vi "列表.vi"(9 "Bool引用句柄":refnum<vi>, 10 "簇":T4, 11 "事件注册引用句柄 2":refnum<event-registration>) -> ()   [LabVIEW 2020]
uses:
  <vilib>/Utility/miscctls.llb/LVRowAndColumnUnsignedTypeDef.ctl
  <vilib>/Utility/miscctls.llb/LVRectTypeDef.ctl
  Windows/System32/user32.dll
panel:
  in  "布尔 3":T1
  in  "布尔 2":T2
  in  "布尔":T3
  in  "多列列表框":i32(listbox)
  # "所有数据"
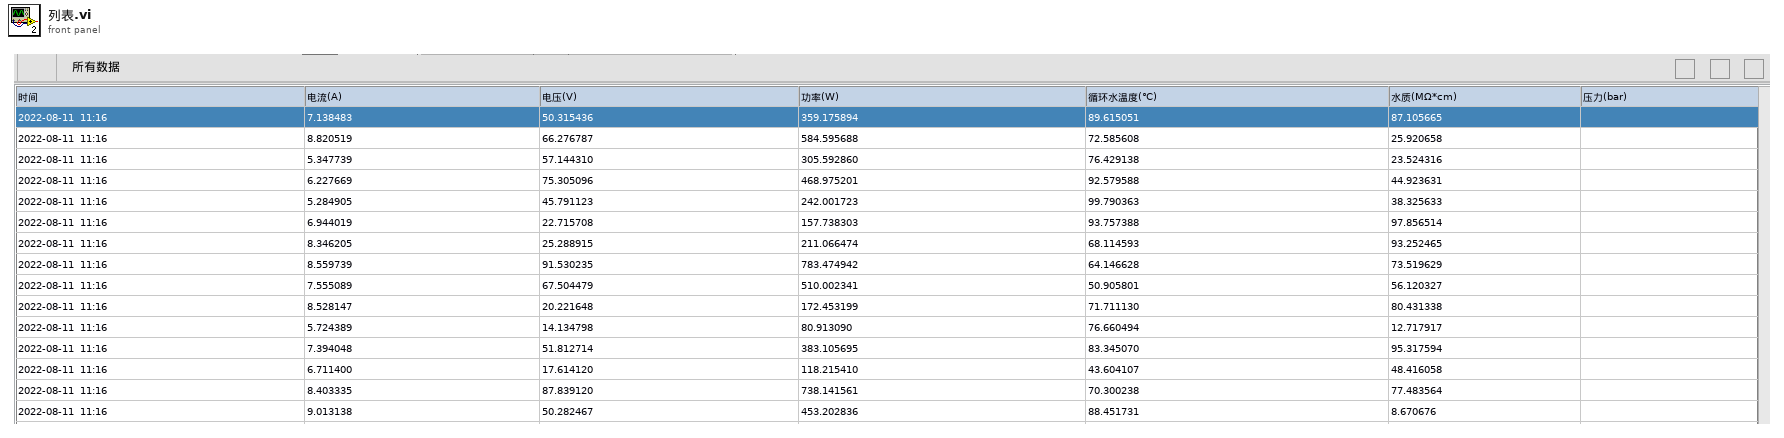
[diagram p1: front panel]
types:
  T1 = typedef "控件关闭.ctl" = bool
  T2 = typedef "控件最小化.ctl" = bool
  T3 = typedef "控件最大化.ctl" = bool
  T4 = cluster{"A1":refnum<vi>, "A2":refnum<vi>, "A3":refnum<vi>, "A4":refnum<vi>}
  T5 = typedef "LVRectTypeDef.ctl" = cluster{"Left":i16, "Top":i16, "Right":i16, "Bottom":i16}
  T6 = typedef "LVRowAndColumnUnsignedTypeDef.ctl" = cluster{"Row":u32, "Column":u32}
  T7 = enum32{"Invalid", "Standard", "Closed", "Hidden", "Minimized", "Maximized"}
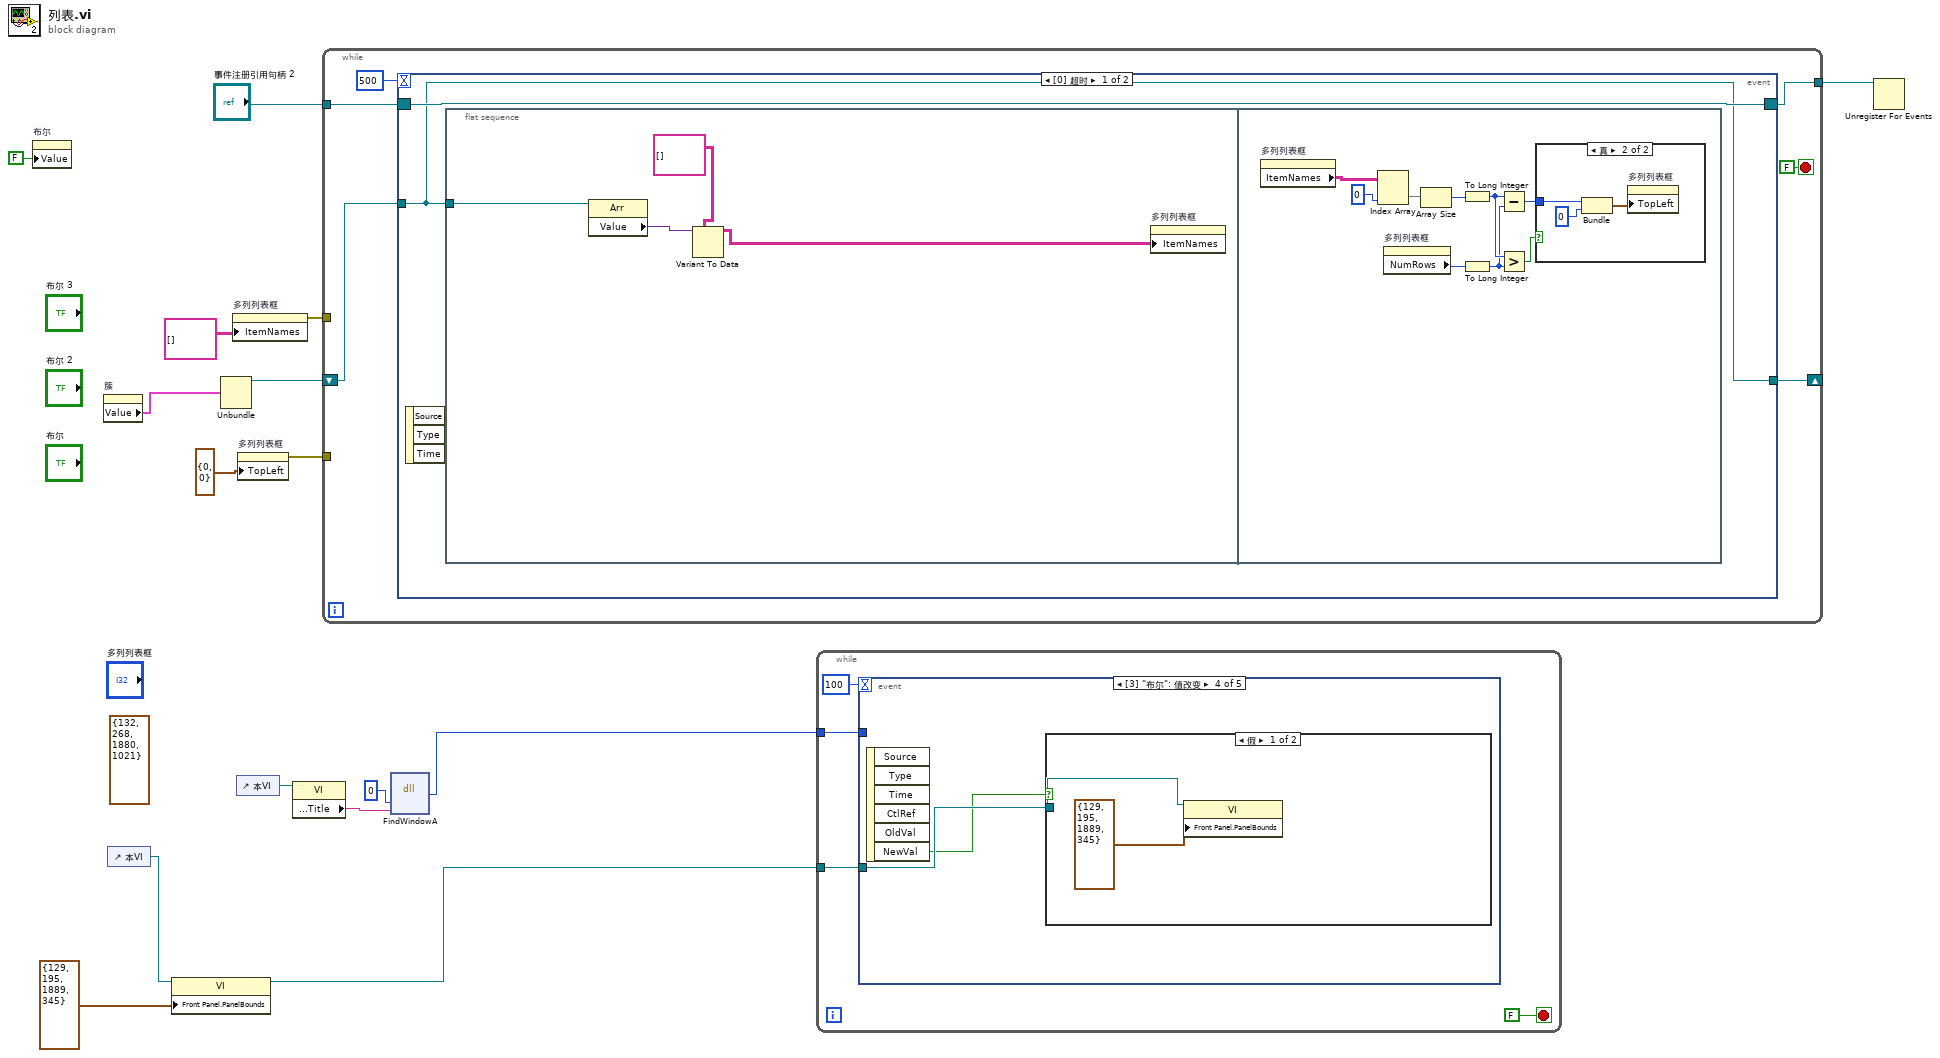
[diagram p0: block diagram]
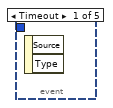
[diagram p2: hidden frame]
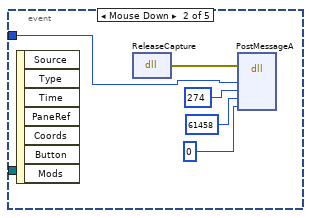
[diagram p3: hidden frame]
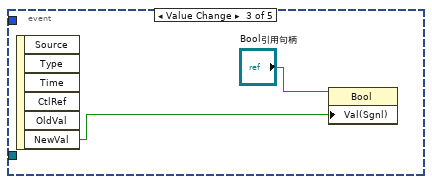
[diagram p4: hidden frame]
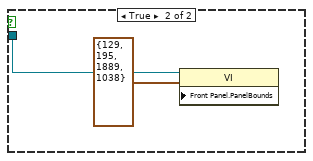
[diagram p5: hidden frame]
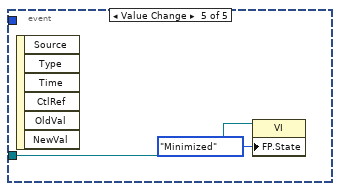
[diagram p6: hidden frame]
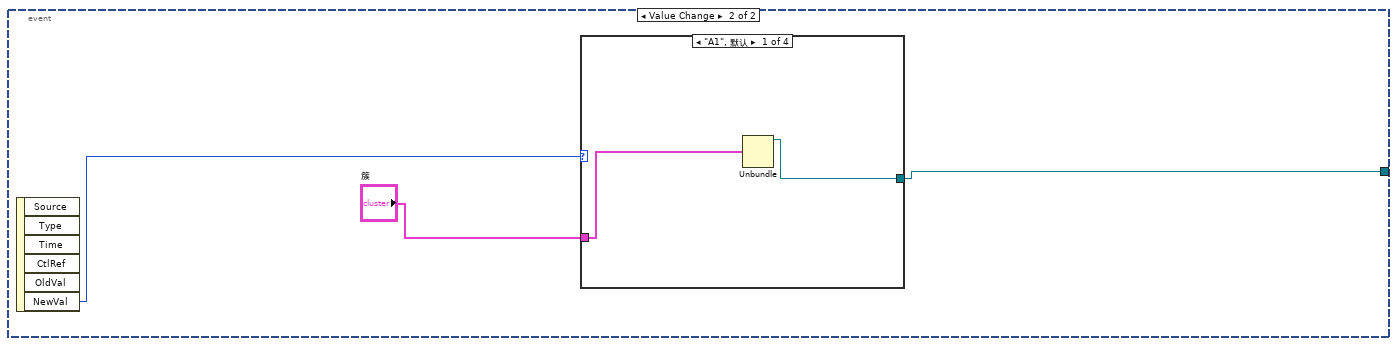
[diagram p8: hidden frame]
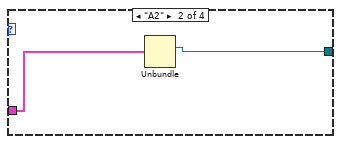
[diagram p9: hidden frame]
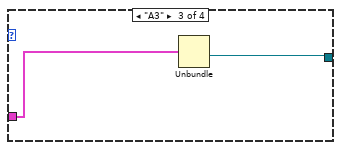
[diagram p10: hidden frame]
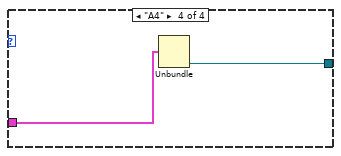
[diagram p11: hidden frame]
diagram:
  (unwired) T5 {"Left"=132, "Top"=268, "Right"=1880, "Bottom"=1021} ("前面板窗口:前面板边界")
  n1 = property on="布尔" class="Bool (严格)"("Value"=T3 FALSE ("布尔")) -> ()  [unwired: 2 in, 2 out]
  n2 = property on="簇" class="Clust (严格)"() -> ("Value"=w3:T4)  [unwired: 2 in, 2 out]
  n3 = control-ref of="本VI"() -> (w14:refnum<vi>)
  n4 = property class="VI"(reference=w14, "Front Panel.PanelBounds"=T5 {"Left"=129, "Top"=195, "Right"=1889, "Bottom"=345} ("前面板窗口:前面板边界")) -> (reference out=w6:refnum<vi>)  [unwired: 1 in, 1 out]
  n5 = Unbundle(w3) -> ("A1"=w2:refnum<vi>)  [unwired: 3 out]
  n6 = property on="多列列表框" class="MCListbox (严格)"("ItemNames"=string[][] []) -> (error out=w16:errorcluster)  [unwired: 2 in, 1 out]
  n7 = control-ref of="本VI"() -> (w12:refnum<vi>)
  n8 = property on="多列列表框" class="MCListbox (严格)"("TopLeft"=T6 {"Row"=0, "Column"=0} ("左上可见单元格")) -> (error out=w10:errorcluster)  [unwired: 2 in, 1 out]
  n9 = property class="VI"(reference=w12) -> ("Front Panel.Title"=w11:string)  [unwired: 1 in, 2 out]
  n10 = while {
    tunnel: w16 -> [_]
    tunnel: w10 -> [_]
    tunnel: "事件注册引用句柄 2" -> [w21]
    tunnel: [w20] -> w4
    shift-right: [w18] -> _
    shift-left: w2 -> [w19]
    stop <- FALSE stop-if-true
    n11 = event shown="[0] 超时" {
      selector: w21 -> [w24 _]
      dyn-events: [w24 _] -> w20
      timeout: 500 -> [_ _]
      tunnel: w19 -> [w23 _]
      tunnel: [w23 w41] -> w18
      event Timeout {
        n12 = event-data() -> ()  [unwired: 1 in, 3 out]
        n13 = flat-sequence {
          tunnel: w23 -> [w26]
          frame #0 {
            n14 = property class="Arr"(reference=w26) -> ("Value"=w28:variant)  [unwired: 1 in, 2 out]
            n15 = Variant To Data(type=string[][] [], Variant=w28) -> (data=w25:string[][])  [unwired: 1 in, 1 out]
            n16 = property on="多列列表框" class="MCListbox (严格)"("ItemNames"=w25) -> ()  [unwired: 2 in, 2 out]
          }
          frame #1 {
            n17 = property on="多列列表框" class="MCListbox (严格)"() -> ("ItemNames"=w37:string[][])  [unwired: 2 in, 2 out]
            n18 = Index Array(array=w37, index (col)=0 ("禁用的索引 (列)")) -> (element=w36:string[])  [unwired: 1 in]
            n19 = property on="多列列表框" class="MCListbox (严格)"() -> ("NumRows"=w33:u32)  [unwired: 2 in, 2 out]
            n20 = Array Size(array=w36) -> (size(s)=w34:i32)
            n21 = To Long Integer(number=w34) -> (32bit integer=w31:i32)
            n22 = To Long Integer(number=w33) -> (32bit integer=w30:i32)
            n23 = Subtract(x=w31, y=w30) -> (x-y=w29:i32)
            n24 = Greater?(x=w31, y=w30) -> (0:w32:bool)
            n25 = case shown="真" w32 {
              tunnel: w29 -> [_ w40]
              frame False {
              }
              frame True {
                n26 = Bundle(w40, 0) -> (w38:cluster{i32, i32})  [unwired: 1 in]
                n27 = property on="多列列表框" class="MCListbox (严格)"("TopLeft"=w38) -> ()  [unwired: 2 in, 2 out]
              }
            }
          }
        }
      }
      event Value Change {
        n28 = event-data() -> ("NewVal"=w42:enum32{"未选择", "A1", "A2", "A3", "A4"})  [unwired: 1 in, 5 out]
        n29 = case shown="\"A1\", 默认" w42 {
          tunnel: "簇" -> [w44 w47 w49 w51]
          tunnel: [w45 w46 w48 w50] -> w41
          frame "A1", Default {
            n30 = Unbundle(w44) -> ("A1"=w45:refnum<vi>)  [unwired: 3 out]
          }
          frame "A2" {
            n31 = Unbundle(w47) -> ("A2"=w46:refnum<vi>)  [unwired: 3 out]
          }
          frame "A3" {
            n32 = Unbundle(w49) -> ("A3"=w48:refnum<vi>)  [unwired: 3 out]
          }
          frame "A4" {
            n33 = Unbundle(w51) -> ("A4"=w50:refnum<vi>)  [unwired: 3 out]
          }
        }
      }
    }
  }
  n34 = dll-call lib="/Windows/System32/user32.dll" fn="FindWindowA"("lp"=u32 0, "name"=w11) -> ("返回类型"=w8:u32)  [unwired: 5 in, 2 out]
  n35 = while {
    tunnel: w8 -> [w55]
    tunnel: w6 -> [w54]
    stop <- FALSE stop-if-true
    n36 = event shown="[3] \"布尔\": 值改变" {
      selector: _ -> [_ _ _ _ _]
      dyn-events: _ -> [_ _ _ _ _]
      timeout: 100 -> [_ _ _ _ _]
      tunnel: w55 -> [_ w56 _ _ _]
      tunnel: w54 -> [_ _ _ w64 w70]
      event Timeout {
        n37 = event-data() -> ()  [unwired: 1 in, 2 out]
      }
      event Mouse Down {
        n38 = event-data() -> ()  [unwired: 1 in, 7 out]
        n39 = dll-call lib="/Windows/System32/user32.dll" fn="ReleaseCapture"() -> (error out=w60:errorcluster)  [unwired: 4 in, 1 out]
        n40 = dll-call lib="/Windows/System32/user32.dll" fn="PostMessageA"(error in=w60, "lp"=w56, "name"=274, "vak"=61458, "val"=0) -> ()  [unwired: 7 in, 2 out]
      }
      event Value Change {
        n41 = event-data() -> ("NewVal"=w61:T1)  [unwired: 1 in, 5 out]
        n42 = property class="Bool"(reference="Bool引用句柄", "Val(Sgnl)"=w61) -> ()  [unwired: 1 in, 2 out]
      }
      event Value Change {
        n43 = event-data() -> ("NewVal"=w63:T3)  [unwired: 1 in, 5 out]
        n44 = case shown="假" w63 {
          tunnel: w64 -> [w65 w68]
          frame False {
            n45 = property class="VI"(reference=w65, "Front Panel.PanelBounds"=T5 {"Left"=129, "Top"=195, "Right"=1889, "Bottom"=345} ("前面板窗口:前面板边界")) -> ()  [unwired: 1 in, 2 out]
          }
          frame True {
            n46 = property class="VI"(reference=w68, "Front Panel.PanelBounds"=T5 {"Left"=129, "Top"=195, "Right"=1889, "Bottom"=1038} ("前面板窗口:前面板边界")) -> ()  [unwired: 1 in, 2 out]
          }
        }
      }
      event Value Change {
        n47 = event-data() -> ()  [unwired: 1 in, 6 out]
        n48 = property class="VI"(reference=w70, "FP.State"=T7."Minimized" ("前面板窗口:状态")) -> ()  [unwired: 1 in, 2 out]
      }
    }
  }
  n49 = Unregister For Events(event registration refnum=w4) -> ()  [unwired: 1 in, 1 out]
